vi "main_hall_effect.vi"() -> ()   [LabVIEW 2018]
uses:
  <instrlib>/Keithley 622x LV 2009/Configure/Source/Typedefs/KE622x -- Current Range.ctl
  <instrlib>/Keithley 622x LV 2009/Configure/Source/Typedefs/KE622x -- Current Ranges.ctl
  <instrlib>/Keithley 622x LV 2009/Typedefs/KE622x -- On Off Control.ctl
  <instrlib>/Keithley 622x LV 2009/Configure/Output/Typedefs/KE6221 -- Output Response.ctl
  <instrlib>/Keithley 622x LV 2009/Configure/Source/Typedefs/KE622x -- Voltage Limit.ctl
  <instrlib>/Keithley 622x LV 2009/Configure/Source/Typedefs/KE622x -- Current Level.ctl
  <instrlib>/Keithley 622x LV 2009/Utility/Typedefs/KE622x -- Instrument Type.ctl
  <vilib>/Analysis/baseanly.llb/Mean (DBL).vi
  <vilib>/Utility/file.llb/Write Delimited Spreadsheet (string).vi
  <instrlib>/Keithley 3706/Keithley 3700 Series.lvlib
  <instrlib>/Keithley 622x LV 2009/Keithley 622x.lvlib
  <vilib>/Analysis/NI_AALBase.lvlib
panel:
  in  "Step Size":dbl format="%#_6f"
  in  "End":dbl format="%#_6e"
  in  "Start":dbl format="%#_6e"
  in  "Rate":dbl=10.0
  in  "Temperature":dbl=300.0
  in  "Approach 2":i32(ring) items=["FastSettle", "NoOvershoot"]
  in  "InstrumentType":i32(ring) items=["PPMS", "VersaLab", "DynaCool", "SVSM", "OptiCool"]
  in  "Remote":bool
  in  "IP Address":string="127.0.0.1"
  out "Chamber\nStatus":i32(ring) items=["ChamberUnknown"=0, "PurgedAndSealed"=1, "VentedAndSealed"=2, "Sealed"=3, "Purging"=4, "Venting"=5, "PreHiVac"=6, "HighVac"=7, "PumpContinuous"=8, "VentContinuous"=9, "ChamberFailure"=15]
  out "Measuring":bool
  out "Temperature\nStatus":i32(ring) items=["TemperatureUnknown"=0, "Stable"=1, "Tracking"=2, "Near"=5, "Chasing"=6, "Filling"=7, "Standby"=10, "Disabled"=13, "ImpedanceNotFunction"=14, "TempFailure"=15]
  out "Field\nStatus":i32(ring) items=["MagnetUnknown"=0, "StablePersistent"=1, "WarmingSwitch"=2, "CoolingSwitch"=3, "StableDriven"=4, "Iterating"=5, "Charging"=6, "Discharging"=7, "CurrentError"=8, "MagnetFailure"=15]
  out "Field 2":dbl
  out "Temperature 2":dbl
  in  "Approach":i32(ring) items=["Linear", "NoOvershoot", "Oscillate"]
  in  "Requested Delay After Stability":dbl=5.0
  in  "Mode":i32(ring) items=["Persistent", "Driven"]
  in  "Field Rate":dbl=100.0
  in  "file path (dialog if empty)":path
  in  "Current Level (A) In":T1=0.1 min=-0.105 max=0.105 format="%.4p"
  out "Current  (A)":dbl
  out "Configuration Error":errorcluster
  in  "Voltage Limit (V)":T2=10.0 min=0.1 max=105.0 step=0.01 format="%.2p"
  in  "Output Response":T3=enum."Slow"
  in  "Analog Filter State":T4
  in  "Current Range In":T5={"Auto Range?"=TRUE, "Man / Selected\nRange"=enum."2nA"}
  in  "Check For SCPI Errors? (T)":bool=TRUE
  in  "VISA resource dc ac current source (16)":refnum<visa-resource-name>
  in  "array":dbl[](array[numeric])
  out "error at Current off":errorcluster
  out "Mean Voltage  (V1-V8)":dbl
  in  "Measure Count (10)":u32=10 min=1
  in  "Function (2: DC Volts)":T7(ring)=enum."DC Volts"
  out "Measurements":dbl[](array[numeric]) format="%#_6e"
  in  "Timeout (30000 milliseconds)":u32=30000
  out "error at current On":errorcluster
  out "Voltage Limit?":bool
  out "Interlock Tripped?":bool
  in  "Turn Off Output If Voltage Limit?":bool=TRUE
  in  "Operation 3":T8(ring)
  in  "Operation 5":T8(ring)
  in  "Unguarded/Guarded":enum32{"UnGuarded", "Guarded"}(radio)
  out "Close Channel List 2":string
  in  "VISA Switch":refnum<visa-resource-name>="GPIB::6"
  # "Switch"
  # "DMM"
  # "TEMPERATURE CONTROL"
  # "FIELD CONTROL"
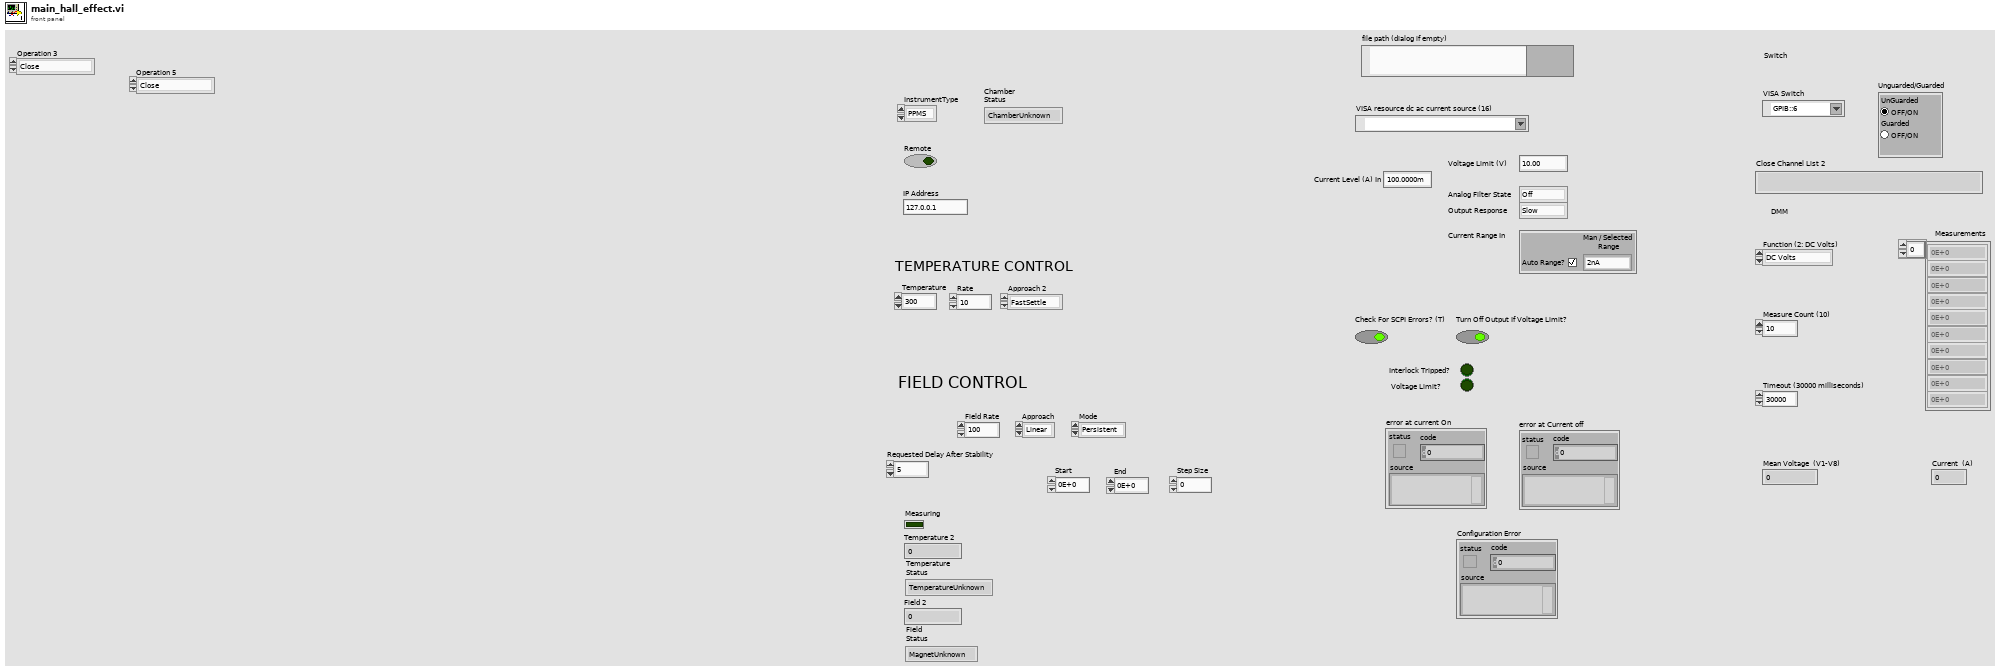
[diagram p1: front panel]
types:
  T1 = typedef "Keithley 622x.lvlib/KE622x -- Current Level.ctl" = dbl
  T2 = typedef "Keithley 622x.lvlib/KE622x -- Voltage Limit.ctl" = dbl
  T3 = typedef "Keithley 622x.lvlib/KE6221 -- Output Response.ctl" = enum16{"Fast", "Slow"}
  T4 = typedef "Keithley 622x.lvlib/KE622x -- On Off Control.ctl" = enum16{"Off", "On"}
  T5 = typedef "Keithley 622x.lvlib/KE622x -- Current Range.ctl" = cluster{"Auto Range?":bool, "Man / Selected\nRange":T6}
  T6 = typedef "Keithley 622x.lvlib/KE622x -- Current Ranges.ctl" = enum16{"2nA", "20nA", "200nA", "2uA", "20uA", "200uA", "2mA", "20mA", "100mA"}
  T7 = enum16{"None", "DC Volts", "AC Volts", "DC Current", "AC Current", "2-Wire Ohms", "4-Wire Ohms", "Temperature", "Period", "Frequency", "Continuity", "Commonside Ohms"}
  T8 = enum16{"Close", "Close Exclusive", "Close Slot Exclusive", "Open", "Open All"}
  T9 = typedef "Keithley 622x.lvlib/KE622x -- Instrument Type.ctl" = enum16{"KE6220", "KE6221"}
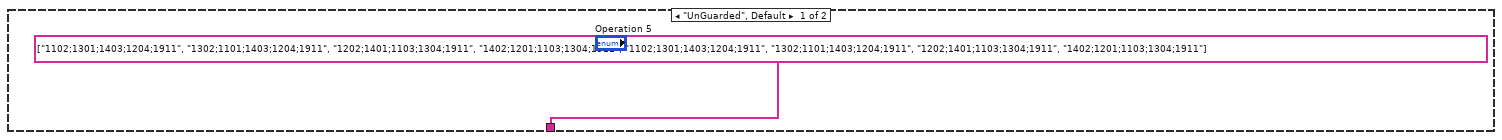
[diagram p3: hidden frame]
diagram:
  n1 = flat-sequence {
    tunnel: [w12] -> w10
    tunnel: [w11] -> w9
    tunnel: w10 -> [w37]
    tunnel: w9 -> [w36]
    tunnel: [w37] -> w8
    tunnel: [w36] -> w7
    tunnel: w3 -> [w35]
    tunnel: "Step Size" -> [w34]
    tunnel: "Start" -> [w33]
    tunnel: w8 -> [w205]
    tunnel: w7 -> [w204]
    frame #0 {
      w26 = 1 items=["Seal", "PurgeAndSeal", "VentAndSeal", "PumpContinuous", "VentContinuous", "HighVacuum"] ("Code")
      n2 = call "OpenQDInstrument.vi"("Remote"="Remote", "IP Address"="IP Address", "InstrumentType"="InstrumentType") -> ("error out"=w23:errorcluster, "Instrument Ref"=w32:refnum<k24>)  [unwired: 5 in]
      n3 = call "SetChamber.vi"("Code"=w26, "error in (no error)"=w23, "Instrument Ref In"=w32) -> ("error out"=w24:errorcluster, "Instrument Ref Out"=w21:refnum<k24>)  [unwired: 1 out]
      n4 = call "WaitFor.vi"("Wait For Chamber"=TRUE ("WaitForChamber"), "Wait For Position"=FALSE ("WaitForPosition"), "Wait For Field"=FALSE ("WaitForField"), "Wait For Temperature"=FALSE ("WaitForTemperature"), "error in (no error)"=w24, "Instrument Ref In"=w21) -> ("error out"=w25:errorcluster, "Instrument Ref Out"=w22:refnum<k24>)  [unwired: 4 in]
      n5 = call "GetChamber.vi"("error in (no error)"=w25, "Instrument Ref In"=w22) -> ("Chamber\nStatus"=→"Chamber\nStatus":i32, "error out"=w14:errorcluster, "Instrument Ref Out"=w13:refnum<k24>)  [unwired: 2 in, 1 out]
      n6 = call "SetTemperature.vi"("Approach"="Approach 2", "Rate"="Rate", "Temperature"="Temperature", "error in (no error)"=w14, "Instrument Ref In"=w13) -> ("error out"=w11:errorcluster, "Instrument Ref Out"=w12:refnum<k24>)  [unwired: 2 in, 1 out]
    }
    frame #1 {
      n7 = for {
        N: w35 -> [_]
        tunnel: w37 -> [w44]
        tunnel: w36 -> [w43]
        tunnel: w34 -> [w39]
        tunnel: w33 -> [w38]
        i -> [w40]
        n8 = flat-sequence {
          tunnel: w44 -> [w53]
          tunnel: w43 -> [w52]
          tunnel: [w51] -> w42
          tunnel: [w50] -> w41
          tunnel: w40 -> [w49]
          tunnel: w39 -> [w48]
          tunnel: w38 -> [w46]
          tunnel: w42 -> [w84]
          tunnel: w41 -> [w83]
          frame #0 {
            n9 = Multiply(x=w48, y=w49) -> (x*y=w47:dbl)
            n10 = Add(x=w46, y=w47) -> (x+y=w45:dbl)
            n11 = call "SetField.vi"("Mode"="Mode", "Approach"="Approach", "Rate"="Field Rate", "Field"=w45, "error in (no error)"=w52, "Instrument Ref In"=w53) -> ("error out"=w64:errorcluster, "Instrument Ref Out"=w65:refnum<k24>)  [unwired: 1 in, 1 out]
            n12 = call "WaitFor.vi"("Delay"="Requested Delay After Stability", "Wait For Field"=TRUE, "Wait For Temperature"=TRUE, "error in (no error)"=w64, "Instrument Ref In"=w65) -> ("error out"=w55:errorcluster, "Instrument Ref Out"=w54:refnum<k24>)  [unwired: 5 in]
            n13 = for {
              N: 20 -> [_]
              shift-right: [w82] -> _
              shift-left: TRUE -> [w80]
              shift-right: [w77] -> _
              shift-left: w55 -> [w79]
              tunnel: w54 -> [w76]
              tunnel: [w74] -> _
              tunnel: [w71] -> w59
              tunnel: [w70] -> w58
              tunnel: [w72] -> w56 mode=indexing
              tunnel: [w73] -> w57 mode=indexing
              n14 = Not(x=w80) -> (.not. x?=w82:bool)
              n15 = local write "Measuring"(w80) -> ()
              n16 = call "GetTemperature.vi"("error in (no error)"=w79, "Instrument Ref In"=w76) -> ("Temperature\nStatus"=w70:i32, "Temperature"=w73:dbl, "error out"=w78:errorcluster, "Instrument Ref Out"=w75:refnum<k24>)  [unwired: 3 in, 1 out]
              n17 = Wait (ms)(milliseconds to wait=u32 200) -> ()  [unwired: 1 out]
              n18 = call "GetField.vi"("error in (no error)"=w78, "Instrument Ref In"=w75) -> ("Field\nStatus"=w71:i32, "Field"=w72:dbl, "error out"=w77:errorcluster, "Instrument Ref Out"=w74:refnum<k24>)  [unwired: 3 in, 1 out]
            }
            "Field\nStatus" <- w59
            "Temperature\nStatus" <- w58
            n19 = call-poly <vilib>:"Mean.vi"("X"=w56) -> ("mean"=w51:dbl)  [unwired: 1 out]
            "Field 2" <- w51
            n20 = call-poly <vilib>:"Mean.vi"("X"=w57) -> ("mean"=w50:dbl)  [unwired: 1 out]
            "Temperature 2" <- w50
          }
          frame #1 {
            n21 = flat-sequence {
              tunnel: [w92] -> w88
              tunnel: [w91] -> w87
              tunnel: [w90] -> w86
              tunnel: ["Current Level (A) In"] -> w85
              tunnel: w88 -> [w135]
              tunnel: w87 -> [w134]
              tunnel: w86 -> [w133]
              tunnel: w85 -> [w132]
              tunnel: w84 -> [w131]
              tunnel: w83 -> [w124]
              frame #0 {
                w93 = KE622x_--_Instrument_Type."KE6221" ("Instrument Type")
                w100 = FALSE ("Read Back Set Values? (T)")
                # "Set the voltage limit\n(a.k.a. compliance)."
                # "Set the current range\nand level."
                # "With the analog filter enabled,\nthe response time (settling time)\nof the output is slowed down.  How\nmuch it is slowed down depends\non the load impedance."
                n22 = call <instrlib>:"Initialize.vi"("VISA resource name"="VISA resource dc ac current source (16)", "Error Queue Option"=enum16{"Clear Error Queue", "Error Query"}."Clear Error Queue", "Instrument Type"=w93) -> ("VISA resource name out"=w109:refnum<visa-resource-name>, "error out"=w108:errorcluster)  [unwired: 11 in]
                n23 = call <instrlib>:"KE622x -- Set Analog Filter State.vi"("Resource In"=w109, "Check For SCPI Errors? (T)"="Check For SCPI Errors? (T)", "Analog Filter State"="Analog Filter State", "error in (no error)"=w108) -> ("Resource Out (dupl)"=w107:refnum<visa-resource-name>, "error out"=w106:errorcluster)  [unwired: 10 in]
                n24 = case shown="\"KE6221\"" w93 {
                  tunnel: w107 -> [w113 w120]
                  tunnel: w106 -> [w112 w118]
                  tunnel: [w113 w117] -> w103
                  tunnel: "Check For SCPI Errors? (T)" -> [w114 w116]
                  tunnel: [w114 w116] -> w90
                  tunnel: [w112 w115] -> w104
                  frame "KE6220" {
                  }
                  frame "KE6221" {
                    # "For the 6221 only, you can speed up the\noutput response as well (output bandwidth\nis now 1MHz).  This increases the output\nresponse, but will also decrease stability."
                    n25 = call <instrlib>:"KE6221 -- Set Output Response.vi"("Resource In"=w120, "Check For SCPI Errors? (T)"=w116, "KE6221 Output Response"="Output Response", "error in (no error)"=w118) -> ("Resource Out (dupl)"=w117:refnum<visa-resource-name>, "error out"=w115:errorcluster)  [unwired: 10 in]
                  }
                }
                n26 = call <instrlib>:"KE622x -- Set Current Range.vi"("Resource In"=w103, "Check For SCPI Errors? (T)"=w90, "Current Range In"="Current Range In", "error in (no error)"=w104, "Read Back Set Values? (T)"=w100) -> ("Resource Out (dupl)"=w102:refnum<visa-resource-name>, "error out"=w101:errorcluster)  [unwired: 8 in, 1 out]
                n27 = call <instrlib>:"KE622x -- Set Current Level.vi"("Resource In"=w102, "Check For SCPI Errors? (T)"=w90, "Current Level (A) In"="Current Level (A) In", "error in (no error)"=w101, "Read Back Set Value? (T)"=w100) -> ("Resource Out (dupl)"=w99:refnum<visa-resource-name>, "error out"=w98:errorcluster)  [unwired: 8 in, 1 out]
                n28 = call <instrlib>:"KE622x -- Set Voltage Limit.vi"("Resource In"=w99, "Check For SCPI Errors? (T)"=w90, "Voltage Limit (V)"="Voltage Limit (V)", "error in (no error)"=w98) -> ("Resource Out (dupl)"=w91:refnum<visa-resource-name>, "error out"=w92:errorcluster)  [unwired: 10 in]
                n29 = call <vilib>:"Simple Error Handler.vi"("error in (no error)"=w92) -> ("error out"=→"Configuration Error":errorcluster)  [unwired: 4 in, 4 out]
                "Current  (A)" <- "Current Level (A) In"
              }
              frame #1 {
                n30 = for {
                  N: 8 -> [_]
                  tunnel: [w147] -> w123 mode=indexing
                  tunnel: w135 -> [w146]
                  tunnel: w134 -> [w145]
                  tunnel: w133 -> [w144]
                  i -> [w149]
                  n31 = flat-sequence {
                    tunnel: w149 -> [w152]
                    tunnel: ["VISA Switch"] -> w148
                    tunnel: w146 -> [w169]
                    tunnel: w145 -> [w168]
                    tunnel: w148 -> [w181]
                    tunnel: [w176] -> w147
                    tunnel: w146 -> [w200]
                    tunnel: w145 -> [w199]
                    tunnel: w144 -> [w198]
                    frame #0 {
                      # "Switch Config."
                      n32 = case shown="\"Guarded\"" "Unguarded/Guarded" {
                        tunnel: [string[] ["1102;1301;1403;1204;1911", "1302;1101;1403;1204;1911", "1202;1401;1103;1304;1911", "1402;1201;1103;1304;1911", "1102;1301;1403;1204;1911", "1302;1101;1403;1204;1911", "1202;1401;1103;1304;1911", "1402;1201;1103;1304;1911"] string[] ["1102,1301,1403,1204,1405,1911", "1302;1101;1403;1204,1405,1911", "1202;1401;1103;1304,1405,1911", "1402;1201;1103;1304,1405,1911", "1102;1301;1403;1204,1405,1911", "1302;1101;1403;1204,1405,1911", "1202;1401;1103;1304,1405,1911", "1402;1201;1103;1304,1405,1911"]] -> w153
                        frame "UnGuarded", Default {
                        }
                        frame "Guarded" {
                        }
                      }
                      n33 = Index Array(array=w153, index=w152) -> (element=w159:string)
                      n34 = call <instrlib>:"ke37xx Initialize.vi"("VISA resource name"="VISA Switch") -> ("VISA resource name out"=w158:refnum<visa-resource-name>, "error out"=w157:errorcluster)  [unwired: 13 in]
                      n35 = call <instrlib>:"ke37xx Close Channels.vi"("VISA Resource Name"=w158, "Channel List"=w159, "Mode (0: Normal)"=enum16{"Normal", "Exclusive", "Slot Exclusive"}."Normal", "error in (no error)"=w157) -> ("VISA Resource Name Out"=w156:refnum<visa-resource-name>, "error out"=w155:errorcluster)  [unwired: 10 in]
                      n36 = call <instrlib>:"ke37xx Get Closed List.vi"("VISA Resource Name"=w156, "Channel List"="allslots", "error in (no error)"=w155) -> ("VISA Resource Name Out"=w162:refnum<visa-resource-name>, "Closed List"=→"Close Channel List 2":string, "error out"=w163:errorcluster)  [unwired: 10 in]
                      n37 = call <instrlib>:"ke37xx Close.vi"("VISA resource name"=w162, "error in (no error)"=w163) -> ("error out"=w161:errorcluster)  [unwired: 13 in]
                      n38 = call <vilib>:"Simple Error Handler.vi"("error in (no error)"=w161) -> ()  [unwired: 1 in, 8 out]
                      n39 = Wait (ms)(milliseconds to wait=u32 2000) -> ()  [unwired: 1 out]
                    }
                    frame #1 {
                      # "Turn on current"
                      n40 = Wait (ms)(milliseconds to wait=u32 2000) -> ()  [unwired: 1 out]
                      n41 = call <instrlib>:"KE622x -- Turn Output On And Check For Errors.vi"("Resource In"=w168, "Turn Off Output If Compliance?"="Turn Off Output If Voltage Limit?", "error in (no error)"=w169) -> ("Interlock Tripped?"=→"Interlock Tripped?":bool, "Compliance?"=→"Voltage Limit?":bool, "error out"=w171:errorcluster)  [unwired: 9 in, 1 out]
                      n42 = call <vilib>:"Simple Error Handler.vi"("error in (no error)"=w171) -> ("error out"=→"error at current On":errorcluster)  [unwired: 4 in, 4 out]
                    }
                    frame #2 {
                      w189 = "MyBuffer" ("Buffer Name")
                      # "Visa Switch"
                      # "Measure Voltages using Internal DMM"
                      n43 = call "Initalized_altered.vi"("VISA Refnum in"=w181) -> ("error out"=w183:errorcluster, "VISA Refnum out"=w184:refnum<visa-resource-name>)  [unwired: 9 in]
                      n44 = call <instrlib>:"ke37xx Configure Measurement.vi"("VISA Resource Name"=w184, "Function (0: None)"="Function (2: DC Volts)", "error in (no error)"=w183) -> ("VISA Resource Name Out"=w194:refnum<visa-resource-name>, "error out"=w193:errorcluster)  [unwired: 11 in]
                      n45 = call <instrlib>:"ke37xx Create Measurement Buffer.vi"("VISA Resource Name"=w194, "Buffer Name"=w189, "Capacity"="Measure Count (10)", "error in (no error)"=w193) -> ("VISA Resource Name Out"=w192:refnum<visa-resource-name>, "error out"=w182:errorcluster)  [unwired: 10 in]
                      n46 = Multiply(x="Measure Count (10)", y=u32 100) -> (x*y=w186:u32)
                      n47 = call <instrlib>:"ke37xx Measure.vi"("VISA Resource Name"=w192, "Buffer Name"=w189, "Measure Count (1)"="Measure Count (10)", "error in (no error)"=w182) -> ("VISA Resource Name Out"=w191:refnum<visa-resource-name>, "error out"=w190:errorcluster)  [unwired: 7 in, 3 out]
                      n48 = call <instrlib>:"ke37xx Read Measurement Buffer.vi"("VISA Resource Name"=w191, "Buffer Name"=w189, "error in (no error)"=w190, "Bytes To Read (1024)"=w186, "Timeout (10 seconds)"="Timeout (30000 milliseconds)") -> ("VISA Resource Name Out"=w197:refnum<visa-resource-name>, "Readings"=w179:dbl[], "error out"=w187:errorcluster)  [unwired: 4 in, 4 out]
                      "Measurements" <- w179
                      n49 = call <instrlib>:"ke37xx Close.vi"("VISA resource name"=w197, "error in (no error)"=w187) -> ("error out"=w196:errorcluster)  [unwired: 13 in]
                      n50 = call <vilib>:"Simple Error Handler.vi"("error in (no error)"=w196) -> ()  [unwired: 1 in, 8 out]
                      n51 = Add Array Elements(numeric array=w179) -> (sum=w180:dbl)
                      n52 = Divide(x=w180, y="Measure Count (10)") -> (x/y=w176:dbl)
                      "Mean Voltage  (V1-V8)" <- w176
                      n53 = Wait (ms)(milliseconds to wait=u32 500) -> ()  [unwired: 1 out]
                    }
                    frame #3 {
                      # "Turn off Current"
                      n54 = call <instrlib>:"KE622x -- Set Output State.vi"("Resource In"=w199, "Check For SCPI Errors? (T)"=w198, "Output State"=KE622x_--_On_Off_Control."Off", "error in (no error)"=w200) -> ("error out"=w201:errorcluster)  [unwired: 10 in, 1 out]
                      n55 = call <vilib>:"Simple Error Handler.vi"("error in (no error)"=w201) -> ("error out"=→"error at Current off":errorcluster)  [unwired: 4 in, 4 out]
                    }
                  }
                }
                n56 = Insert Into Array(array="array", new element #1=w132, new element #2=w131, new element #3=w124, new element #4=w123) -> (w122:dbl[])  [unwired: 1 in]
                n57 = Array Size(array=w122) -> (size(s)=w121:i32)
                n58 = for {
                  N: w121 -> [_]
                  tunnel: w122 -> [w143]
                  tunnel: [w140] -> w125 mode=indexing
                  i -> [w142]
                  n59 = Index Array(array=w143, index=w142) -> (element=w141:dbl)
                  n60 = Number To Fractional String(number=w141, width (-)=i16 10, precision (6)=i16 10) -> (F-format string=w140:string)  [unwired: 1 in]
                }
                n61 = Insert Into Array(array=string[] [], new element=w125) -> (w127:string[])  [unwired: 1 in]
                n62 = call-poly <vilib>:"Write Delimited Spreadsheet.vi"("file path (dialog if empty)"="file path (dialog if empty)", "1D data"=w127, "append to file? (new file:F)"=TRUE, "delimiter (\\t)"="," ("delimiter (\\t)")) -> ()  [unwired: 10 in, 2 out]
              }
            }
          }
        }
      }
    }
    frame #2 {
      w214 = 0 items=["Persistent", "Driven"] ("Mode")
      w213 = 0 items=["Linear", "NoOvershoot", "Oscillate"] ("Approach")
      w208 = 0 items=["FastSettle", "NoOvershoot"] ("Approach")
      n63 = call "SetTemperature.vi"("Approach"=w208, "Rate"=20.0, "Temperature"=300.0, "error in (no error)"=w204, "Instrument Ref In"=w205) -> ("error out"=w210:errorcluster, "Instrument Ref Out"=w209:refnum<k24>)  [unwired: 2 in, 1 out]
      n64 = call "SetField.vi"("Mode"=w214, "Approach"=w213, "Rate"=200.0, "Field"=0.0, "error in (no error)"=w210, "Instrument Ref In"=w209) -> ("error out"=w216:errorcluster, "Instrument Ref Out"=w215:refnum<k24>)  [unwired: 1 in, 1 out]
      n65 = Close Reference(reference=w215, error in (no error)=w216) -> ()  [unwired: 1 out]
    }
  }
  n66 = Subtract(x="End", y="Start") -> (x-y=w5:dbl)
  n67 = Divide(x=w5, y="Step Size") -> (x/y=w4:dbl)
  n68 = Round Toward -Infinity(1:w4) -> (0:w3:dbl)
